vi "Init Hardware.vi"(8 "error in (no error)":errorcluster, 11 "Quantum Design Driver in":refnum<class "Quantum Design Driver.lvclass">) -> (0 "error out":errorcluster, 3 "Quantum Design Driver out":refnum<class "Quantum Design Driver.lvclass">)   [LabVIEW 2021, in "Quantum Design Driver.lvclass"]
uses:
  Quantum Design Driver.lvclass
  C:/GitHub/NHMFL_Core/Libraries/Instruments/Instrument Driver/Instrument Driver.lvclass
  Quantum Design Driver.lvclass/Quantum Design Driver.ctl
  Instrument Driver/Instrument Driver.lvclass/Instrument Driver.ctl
  Instrument Driver/Write Channel names.vi
  Instrument Driver/Write Channel units.vi
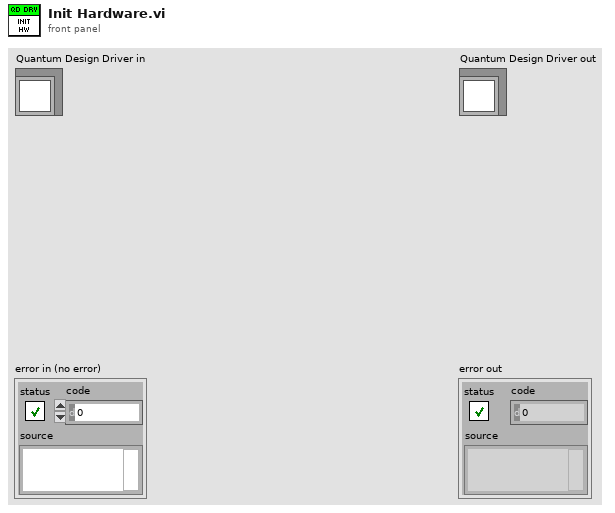
[diagram p1: front panel]
types:
  T1 = typedef "Quantum Desing Configuration.ctl" = cluster{"Address":string, "Instrument type":u16, "Remote":bool, "Measurements":enum16{"Temperature", "Field", "Position"}[]}
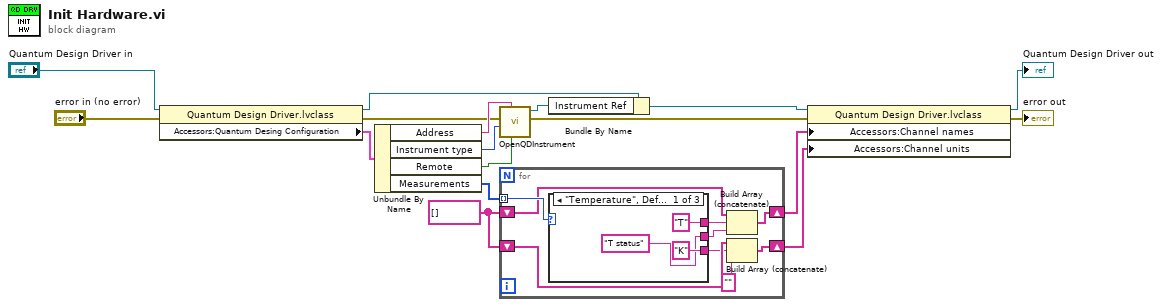
[diagram p0: block diagram]
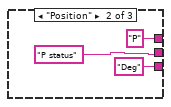
[diagram p2: hidden frame]
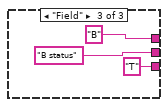
[diagram p3: hidden frame]
diagram:
  w1 = string[] [] ("f")
  n1 = property class="Quantum Design Driver.lvclass"(reference="Quantum Design Driver in", error in="error in (no error)") -> (reference out=w11:refnum<class "Quantum Design Driver.lvclass">, error out=w13:errorcluster, "Accessors:Quantum Desing Configuration"=w15:T1)
  n2 = Unbundle By Name(w15) -> ("Address"=w14:string, "Instrument type"=w12:u16, "Remote"=w8:bool, "Measurements"=w4:enum16{"Temperature", "Field", "Position"}[])
  n3 = call <instrlib>:"OpenQDInstrument.vi"("Remote"=w8, "IP Address"=w14, "Instrument Type"=w12, "error in (no error)"=w13) -> ("error out"=w9:errorcluster, "Instrument Ref"=w10:refnum<k24>)  [unwired: 4 in]
  n4 = for {
    tunnel: w4 -> [w26] mode=indexing
    shift-right: [w23] -> w2
    shift-left: w1 -> [w25]
    shift-right: [w22] -> w3
    shift-left: w1 -> [w21]
    n5 = case shown="\"Temperature\", Default" w26 {
      tunnel: ["K" "Deg" "T"] -> w24
      tunnel: ["T" "P" "B"] -> w20
      tunnel: ["T status" "P status" "B status"] -> w19
      frame "Temperature", Default {
      }
      frame "Position" {
      }
      frame "Field" {
      }
    }
    n6 = Build Array (concatenate)(w21, w20, w19) -> (w22:string[])
    n7 = Build Array (concatenate)(w25, w24, "" ("element")) -> (w23:string[])
  }
  n8 = Bundle By Name(cluster=w11, "Instrument Ref"=w10) -> (w6:refnum<class "Quantum Design Driver.lvclass">)
  n9 = property class="Quantum Design Driver.lvclass"(reference=w6, error in=w9, "Accessors:Channel names"=w3, "Accessors:Channel units"=w2) -> (reference out=→"Quantum Design Driver out":refnum<class "Quantum Design Driver.lvclass">, error out=→"error out":errorcluster)
